vi "Arduino-Listen-RS232-Mantoles-Mod-04-10-2021-REV1.vi"(0 "VISA resource name":refnum<visa-resource-name>, 11 "error in":errorcluster) -> (4 "read buffer":string, 15 "error out":errorcluster)   [LabVIEW 2020]
uses:
  <vilib>/Instr/_visa.llb/VISA Set IO Buffer Mask.ctl
  <vilib>/Instr/_visa.llb/VISA Flush IO Buffer Mask.ctl
  <vilib>/Instr/_visa.llb/VISA Configure Serial Port (Instr).vi
panel:
  out "return count":u32
  in  "data bits (8)":u16=8 min=5 max=8 step=1
  in  "baud rate (115200)":u32=115200
  in  "stop":bool
  # "Working off of this example: \nhttps://microcontrollerslab.com/arduino-labview-data-serial-communication/"
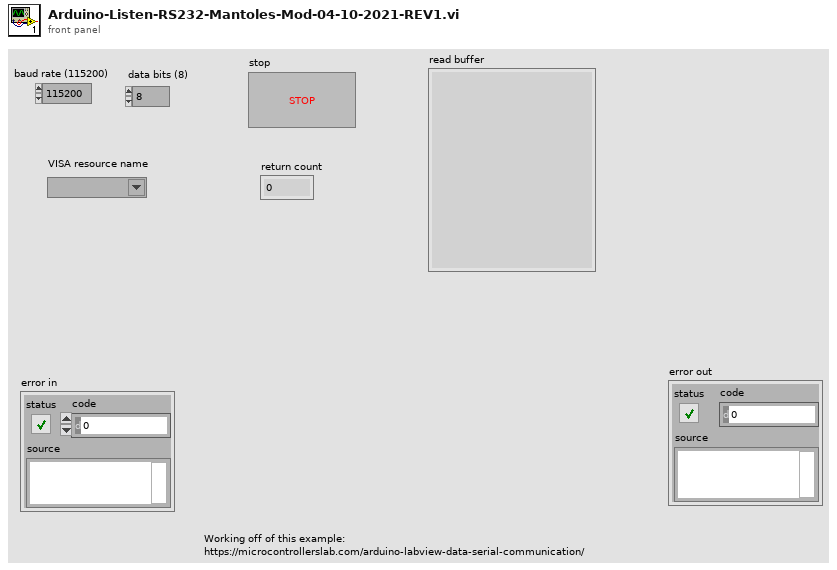
[diagram p1: front panel]
types:
  T1 = typedef "VISA Flush IO Buffer Mask.ctl" = u16
  T2 = typedef "VISA Set IO Buffer Mask.ctl" = u16
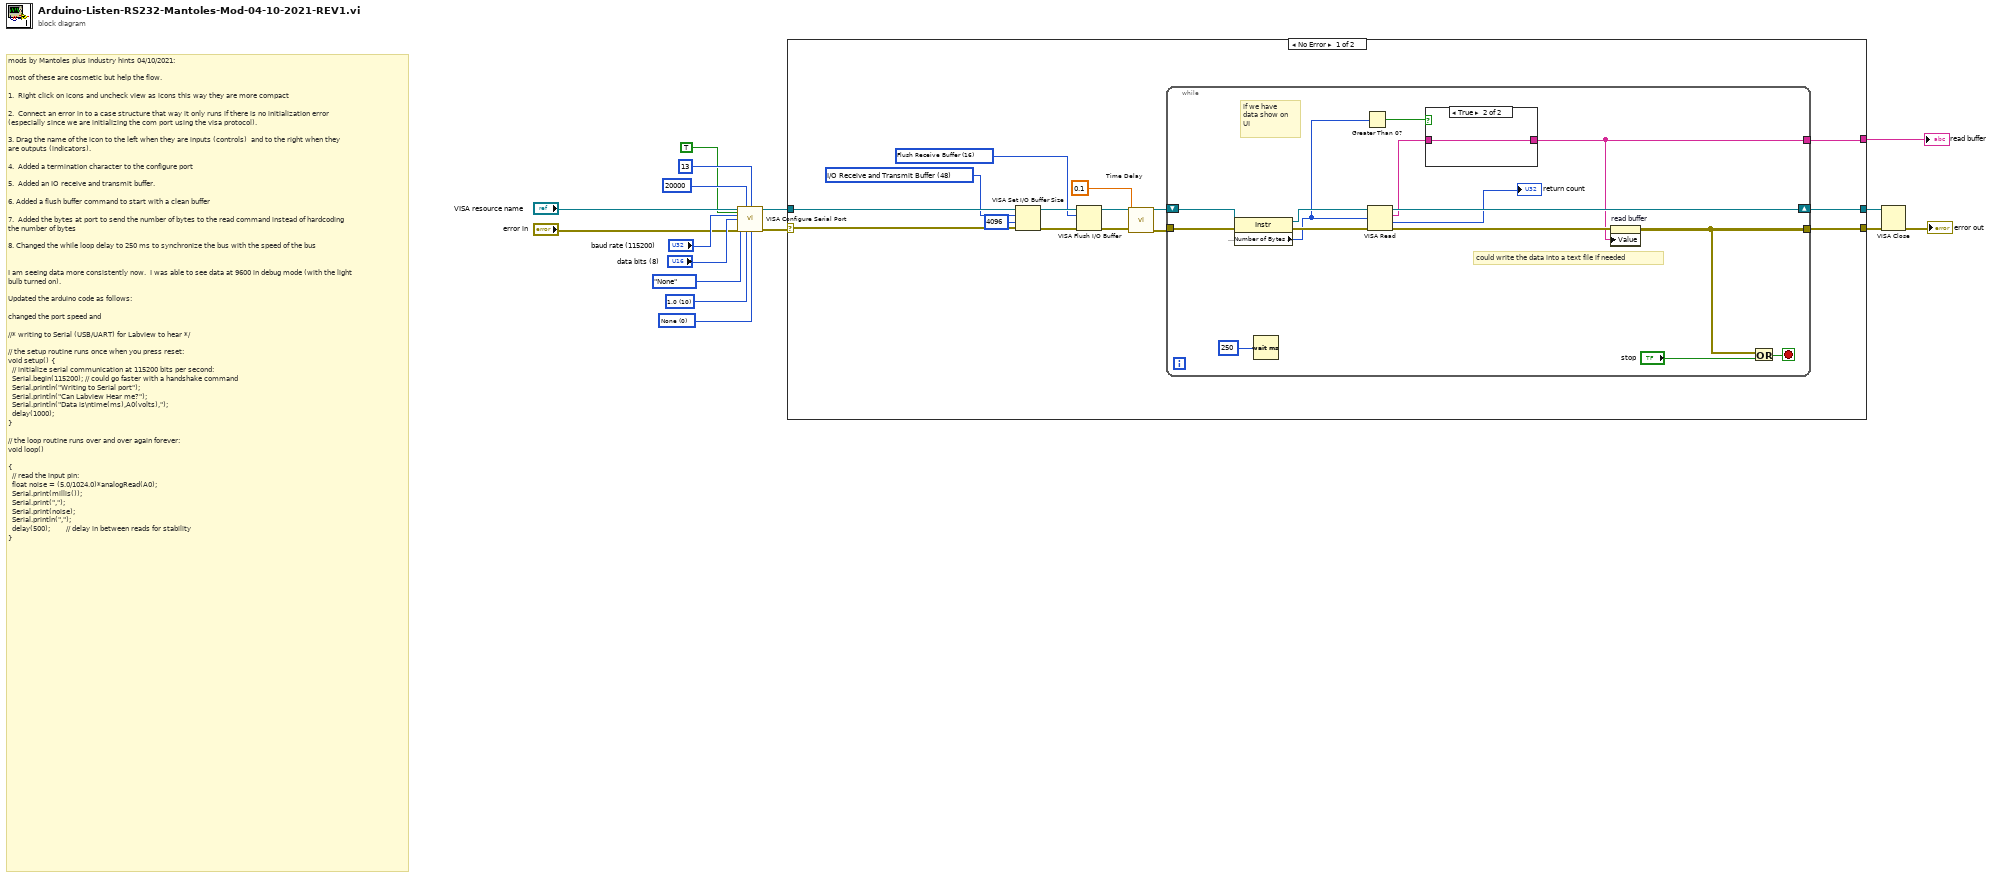
[diagram p0: block diagram]
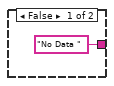
[diagram p2: hidden frame]
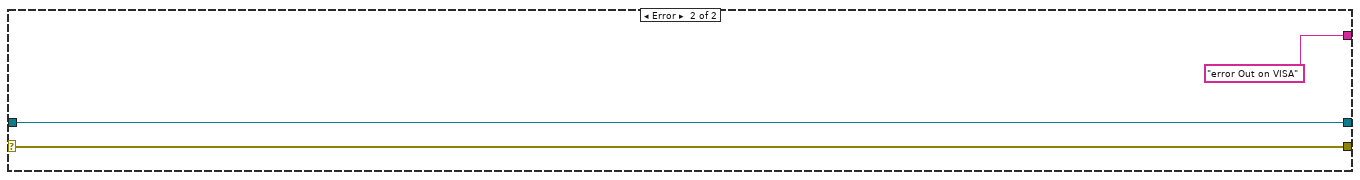
[diagram p3: hidden frame]
diagram:
  w4 = u16 0 items=["None", "XON/XOFF", "RTS/CTS", "XON/XOFF & RTS/CTS", "DTR/DSR", "XON/XOFF & DTR/DSR"] ("flow control (0:none)")
  w5 = u16 10 items=["1.0"=10, "1.5"=15, "2.0"=20] ("stop bits (10: 1 bit)")
  # "mods by Mantoles plus industry hints 04/10/2021:\n\nmost of these are cosmetic but help the flow.\n\n1.  Right click on icons and uncheck view as icons this way they are more compact\n\n2.  Connect an error in to a case structure that way it only runs if there is no initialization error (especially since we are initializing the com port using the visa protocol).\n\n3. Drag the name of the icon to the left when they are inputs (controls)  and to the right when they are outputs (indicators). \n\n4.  Added a termination character to the configure port \n\n5.  Added an IO receive and transmit buffer. \n\n6. Added a flush buffer command to start with a clean buffer\n\n7.  Added the bytes at port to send the number of bytes to the read command instead of hardcoding the number of bytes \n\n8. Changed the while loop delay to 250 ms to synchronize the bus with the speed of the bus\n\n\nI am seeing data more consistently now.  I was able to see data at 9600 in debug mode (with the light bulb turned on).   \n\nUpdated the arduino code as follows:\n\nchanged the port speed and \n\n//* writing to Serial (USB/UART) for Labview to hear */\n\n// the setup routine runs once when you press reset:\nvoid setup() {\n  // initialize serial communication at 115200 bits per second:\n  Serial.begin(115200); // could go faster with a handshake command\n  Serial.println(\"Writing to Serial port\");\n  Serial.println(\"Can Labview Hear me?\");\n  Serial.println(\"Data is\\ntime(ms),A0(volts),\");\n  delay(1000);\n}\n\n// the loop routine runs over and over again forever:\nvoid loop() \n\n{\n  // read the input pin:\n  float noise = (5.0/1024.0)*analogRead(A0);\n  Serial.print(millis());\n  Serial.print(\",\");\n  Serial.print(noise);\n  Serial.println(\",\");\n  delay(500);        // delay in between reads for stability\n}"
  n1 = call-poly "VISA Configure Serial Port"("VISA resource name"="VISA resource name", "timeout (10sec)"=u32 20000, "termination char\n(0xA = '\\n' = LF)"=u8 13 ("termination char\n(0xA = '\\n' = LF)"), "Enable Termination\nChar (T)"=TRUE ("Enable Termination\nChar (T)"), "baud rate (9600)"="baud rate (115200)", "data bits (8)"="data bits (8)", "parity (0:none)"=enum16{"None", "Odd", "Even", "Mark", "Space"}."None", "error in (no error)"="error in", "stop bits (10: 1 bit)"=w5, "flow control (0:none)"=w4) -> ("VISA resource name out"=w15:refnum<visa-resource-name>, "error out"=w1:errorcluster)  [unwired: 4 in]
  n2 = case shown="No Error" w1 {
    selector: w1 -> [w18 w48]
    tunnel: [w30 w49] -> w16
    tunnel: [w17 "error Out on VISA" ("read buffer")] -> w11
    tunnel: w15 -> [w26 w49]
    tunnel: [w29 w48] -> w10
    frame No Error {
      w19 = T1 16 items=["Flush Receive Buffer"=16, "Write Transmit Buffer to Device"=32, "Flush Receive Buffer (No I/O)"=64, "Flush Transmit Buffer"=128] ("Mask")
      w25 = T2 48 items=["I/O Receive Buffer"=16, "I/O Transmit Buffer"=32, "I/O Receive and Transmit Buffer"=48] ("Mask")
      n3 = VISA Set I/O Buffer Size(VISA resource name=w26, mask (16)=w25, size (4096)=u32 4096, error in (no error)=w18) -> (VISA resource name out=w27:refnum<visa-resource-name>, error out=w28:errorcluster)
      n4 = VISA Flush I/O Buffer(VISA resource name=w27, mask (16)=w19, error in (no error)=w28) -> (VISA resource name out=w23:refnum<visa-resource-name>, error out=w21:errorcluster)
      n5 = call "Time Delay"("error in (no error)"=w21, "Delay Time (s)"=0.1) -> ("error out"=w20:errorcluster)  [unwired: 9 in]
      n6 = while {
        tunnel: [w33] -> w29
        shift-right: [w45] -> w30
        shift-left: w23 -> [w41]
        tunnel: [w34] -> w17
        tunnel: w20 -> [w40]
        stop <- w43 stop-if-true
        # "could write the data into a text file if needed"
        # "if we have \ndata show on\nUI"
        n7 = property class="Instr"(reference=w41, error in=w40) -> (reference out=w39:refnum<visa-resource-name>, error out=w38:errorcluster, "Serial Settings:Number of Bytes at Serial Port"=w31:u32)
        n8 = Wait (ms)(milliseconds to wait=u32 250) -> ()  [unwired: 1 out]
        n9 = Greater Than 0?(x=w31) -> (x > 0?=w32:bool)
        n10 = VISA Read(VISA resource name=w39, byte count=w31, error in (no error)=w38) -> (VISA resource name out=w45:refnum<visa-resource-name>, read buffer=w36:string, return count=→"return count":u32, error out=w35:errorcluster)
        n11 = case shown="True" w32 {
          tunnel: w36 -> [_ w47]
          tunnel: ["No Data " ("read buffer") w47] -> w34
          frame False {
          }
          frame True {
          }
        }
        n12 = property on="read buffer" class="Str"(error in=w35, "Value"=w34) -> (error out=w33:errorcluster)  [unwired: 1 in, 1 out]
        n13 = Or(x=w33, y="stop") -> (x .or. y?=w43:bool)
      }
    }
    frame Error {
    }
  }
  "read buffer" <- w11
  n14 = VISA Close(VISA resource name=w16, error in (no error)=w10) -> (error out=→"error out":errorcluster)
